vi "Read register Info.vi"() -> ()   [LabVIEW 2011]
uses:
  <vilib>/registry/registry.llb/Registry RtKey.ctl
  <vilib>/registry/registry.llb/Read Registry Value Simple STR.vi
panel:
  out "value1":string
  out "value2":string
  out "value3":string
  out "values":string[](array[string])
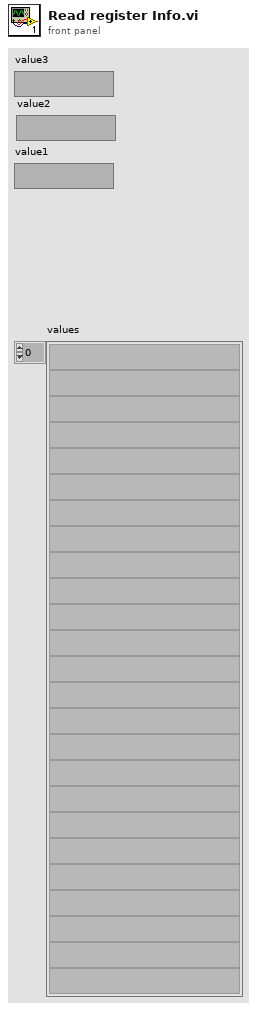
[diagram p1: front panel]
types:
  T1 = typedef "Registry RtKey.ctl" = enum32{"HKEY_CLASSES_ROOT", "HKEY_CURRENT_USER", "HKEY_LOCAL_MACHINE", "HKEY_USERS", "HKEY_PERFORMANCE_DATA", "HKEY_CURRENT_CONFIG", "HKEY_DYN_DATA"}
  T2 = typedef "Registry refnum.ctl" = refnum<k1>
  T3 = cluster{"numValues":i32, "maxValueNameLen":i32, "maxValueDataLen":i32}
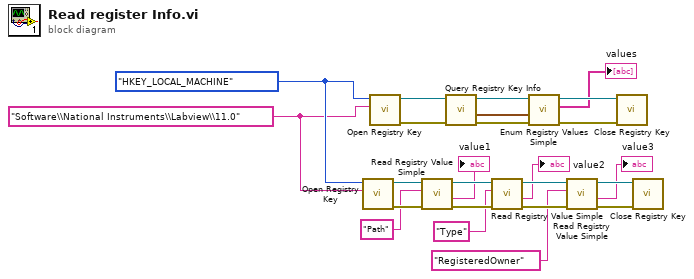
[diagram p0: block diagram]
diagram:
  w7 = "Software\\National Instruments\\Labview\\11.0" ("subkey")
  w8 = Registry_RtKey."HKEY_LOCAL_MACHINE" ("root key (HKEY_LOCAL_MACHINE)")
  n1 = call <vilib>:"Open Registry Key.vi"("subkey"=w7, "root key (HKEY_LOCAL_MACHINE)"=w8) -> ("error out"=w12:errorcluster, "refnum out"=w16:T2)  [unwired: 8 in]
  n2 = call <vilib>:"Open Registry Key.vi"("subkey"=w7, "root key (HKEY_LOCAL_MACHINE)"=w8) -> ("error out"=w23:errorcluster, "refnum out"=w24:T2)  [unwired: 8 in]
  n3 = call-poly <vilib>:"Read Registry Value Simple.vi"("error in (no error)"=w12, "value"="Path" ("subkey"), "refnum"=w16) -> ("error out"=w11:errorcluster, "String/Binary data"=→"value1":string, "refnum out"=w15:T2)  [unwired: 3 in, 1 out]
  n4 = call <vilib>:"Query Registry Key Info.vi"("error in (no error)"=w23, "refnum"=w24) -> ("error out"=w22:errorcluster, "value info"=w17:T3, "refnum out"=w21:T2)  [unwired: 5 in, 2 out]
  n5 = call-poly <vilib>:"Read Registry Value Simple.vi"("error in (no error)"=w11, "value"="Type" ("subkey"), "refnum"=w15) -> ("error out"=w10:errorcluster, "String/Binary data"=→"value2":string, "refnum out"=w14:T2)  [unwired: 3 in, 1 out]
  n6 = call <vilib>:"Enum Registry Values Simple.vi"("error in (no error)"=w22, "value info"=w17, "refnum"=w21) -> ("error out"=w19:errorcluster, "values"=→"values":string[], "refnum out"=w20:T2)  [unwired: 3 in, 3 out]
  n7 = call-poly <vilib>:"Read Registry Value Simple.vi"("error in (no error)"=w10, "value"="RegisteredOwner" ("subkey"), "refnum"=w14) -> ("error out"=w9:errorcluster, "String/Binary data"=→"value3":string, "refnum out"=w13:T2)  [unwired: 3 in, 1 out]
  n8 = call <vilib>:"Close Registry Key.vi"("error in (no error)"=w19, "refnum"=w20) -> ()  [unwired: 5 in, 1 out]
  n9 = call <vilib>:"Close Registry Key.vi"("error in (no error)"=w9, "refnum"=w13) -> ()  [unwired: 5 in, 1 out]
